vi "PLC.Dial750, Read PLC Data.vi"(8 "error in (no error)":errorcluster, 9 "Var Names":string[][](array[string]), 10 "PLC Vars In":T1, 11 "Session Ref":u32) -> (0 "error out":errorcluster, 2 "PLC Variables":T1, 3 "Session Ref Out":u32)   [LabVIEW 2018]
uses:
  Controls/PLC.750 Variables.ctl
  <instrlib>/_Ackermann Automation/TwinCAT ADS Library/TcAdsLV_TCP/TcAdsLV_TCP_3.lvlib
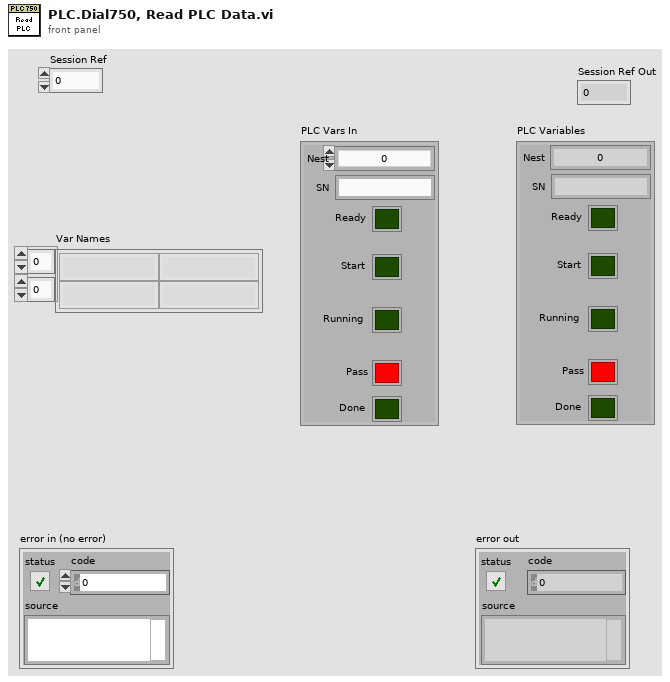
[diagram p1: front panel]
types:
  T1 = typedef "PLC.750 Variables.ctl" = cluster{"Nest":i32, "SN":string, "Ready":bool, "Start":bool, "Pass":bool, "Done":bool, "Running":bool}
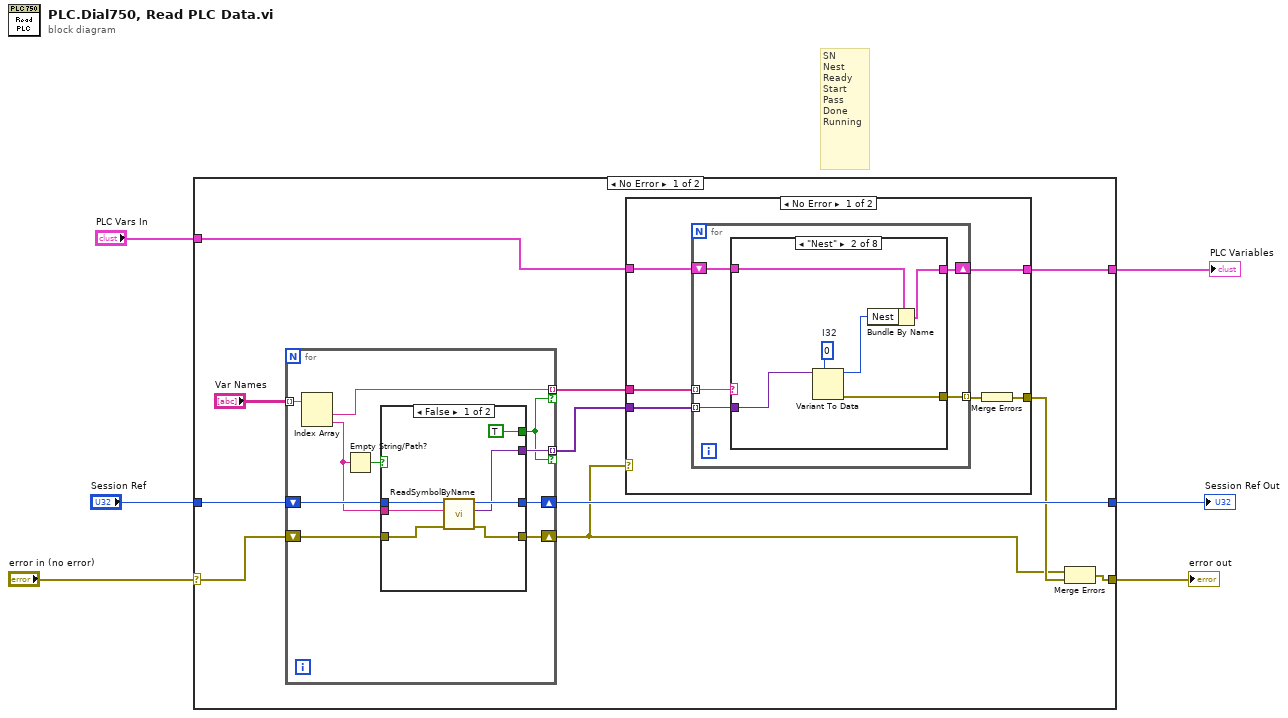
[diagram p0: block diagram]
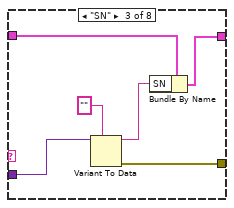
[diagram p3: hidden frame]
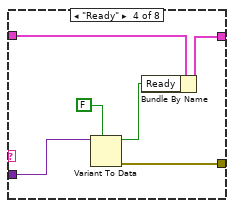
[diagram p4: hidden frame]
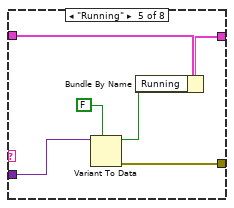
[diagram p5: hidden frame]
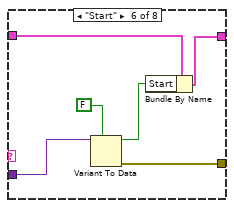
[diagram p6: hidden frame]
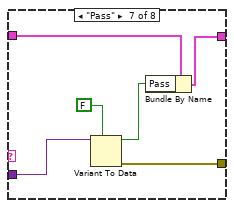
[diagram p7: hidden frame]
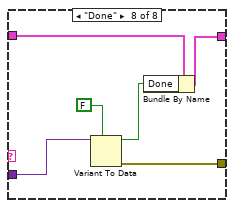
[diagram p8: hidden frame]
diagram:
  # "SN\nNest\nReady\nStart\nPass\nDone\nRunning"
  n1 = case shown="No Error" "error in (no error)" {
    selector: "error in (no error)" -> [w15 w94]
    tunnel: [w7 w94] -> w5
    tunnel: "Session Ref" -> [w17 w93]
    tunnel: [w16 w93] -> w3
    tunnel: "PLC Vars In" -> [w14 w92]
    tunnel: [w12 w92] -> w1
    frame No Error {
      n2 = for {
        tunnel: "Var Names" -> [w78] mode=indexing
        shift-right: [w81] -> w16
        shift-left: w17 -> [w82]
        shift-right: [w80] -> w8
        shift-left: w15 -> [w73]
        tunnel: [w79] -> w11 mode=indexing if=w76
        tunnel: [w77] -> w13 mode=indexing if=w76
        n3 = Index Array(array=w78) -> (element #1=w77:string, element #2=w75:string)  [unwired: 2 in]
        n4 = Empty String/Path?(string/path=w75) -> (empty?=w74:bool)
        n5 = case shown="False" w74 {
          tunnel: w82 -> [w89 w91]
          tunnel: [w88 w91] -> w81
          tunnel: [w87 w90] -> w80
          tunnel: [w86 _] -> w79
          tunnel: w75 -> [w85 _]
          tunnel: [TRUE _] -> w76
          tunnel: w73 -> [w83 w90]
          frame False {
            n6 = call <instrlib>:"ReadSymbolByName.vi"("error in"=w83, "Name"=w85, "Session Ref"=w89) -> ("error out"=w87:errorcluster, "Data"=w86:variant, "Session Ref out"=w88:u32)  [unwired: 3 in, 3 out]
          }
          frame True {
          }
        }
      }
      n7 = case shown="No Error" w8 {
        tunnel: w14 -> [w22 w72]
        tunnel: w13 -> [w23 _]
        tunnel: [w21 w72] -> w12
        tunnel: w11 -> [w20 _]
        tunnel: [w18 _] -> w9
        frame No Error {
          n8 = for {
            tunnel: w23 -> [w27] mode=indexing
            shift-right: [w26] -> w21
            shift-left: w22 -> [w28]
            tunnel: w20 -> [w25] mode=indexing
            tunnel: [w24] -> w19 mode=indexing
            n9 = case shown="\"Nest\"" w27 {
              tunnel: w28 -> [w29 w35 w41 w47 w53 w59 w65 w71]
              tunnel: [w29 w34 w40 w46 w52 w58 w64 w70] -> w26
              tunnel: w25 -> [_ w32 w39 w45 w51 w57 w63 w69]
              tunnel: [_ w30 w36 w42 w48 w54 w60 w66] -> w24
              frame Default {
              }
              frame "Nest" {
                w33 = 0  # I32
                n10 = Variant To Data(type=w33, Variant=w32) -> (data=w31:i32, error out=w30:errorcluster)  [unwired: 1 in]
                n11 = Bundle By Name(cluster=w35, "Nest"=w31) -> (w34:T1)
              }
              frame "SN" {
                n12 = Variant To Data(type="", Variant=w39) -> (data=w38:string, error out=w36:errorcluster)  [unwired: 1 in]
                n13 = Bundle By Name(cluster=w41, "SN"=w38) -> (w40:T1)
              }
              frame "Ready" {
                n14 = Variant To Data(type=FALSE, Variant=w45) -> (data=w44:bool, error out=w42:errorcluster)  [unwired: 1 in]
                n15 = Bundle By Name(cluster=w47, "Ready"=w44) -> (w46:T1)
              }
              frame "Running" {
                n16 = Variant To Data(type=FALSE, Variant=w51) -> (data=w50:bool, error out=w48:errorcluster)  [unwired: 1 in]
                n17 = Bundle By Name(cluster=w53, "Running"=w50) -> (w52:T1)
              }
              frame "Start" {
                n18 = Variant To Data(type=FALSE, Variant=w57) -> (data=w56:bool, error out=w54:errorcluster)  [unwired: 1 in]
                n19 = Bundle By Name(cluster=w59, "Start"=w56) -> (w58:T1)
              }
              frame "Pass" {
                n20 = Variant To Data(type=FALSE, Variant=w63) -> (data=w62:bool, error out=w60:errorcluster)  [unwired: 1 in]
                n21 = Bundle By Name(cluster=w65, "Pass"=w62) -> (w64:T1)
              }
              frame "Done" {
                n22 = Variant To Data(type=FALSE, Variant=w69) -> (data=w68:bool, error out=w66:errorcluster)  [unwired: 1 in]
                n23 = Bundle By Name(cluster=w71, "Done"=w68) -> (w70:T1)
              }
            }
          }
          n24 = Merge Errors(w19) -> (w18:errorcluster)
        }
        frame Error {
        }
      }
      n25 = Merge Errors(w8, w9) -> (w7:errorcluster)
    }
    frame Error {
    }
  }
  "error out" <- w5
  "PLC Variables" <- w1
  "Session Ref Out" <- w3
